vi "Add Device to Stack.vi"(8 "error in (no error)":errorcluster, 10 "Device in":refnum<class "Device.lvclass">, 11 "IP Connection in":refnum<class "IP Connection.lvclass">) -> (0 "error out":errorcluster, 2 "Device out":refnum<class "Device.lvclass">, 3 "IP Connection out":refnum<class "IP Connection.lvclass">)   [LabVIEW 2011, in "Tinkerforge.lvlib" / "IP Connection.lvclass"]
doc: "This VI adds <B>Device</B> to the stack."
uses:
  IP Connection.lvclass
  Device/Device.lvclass
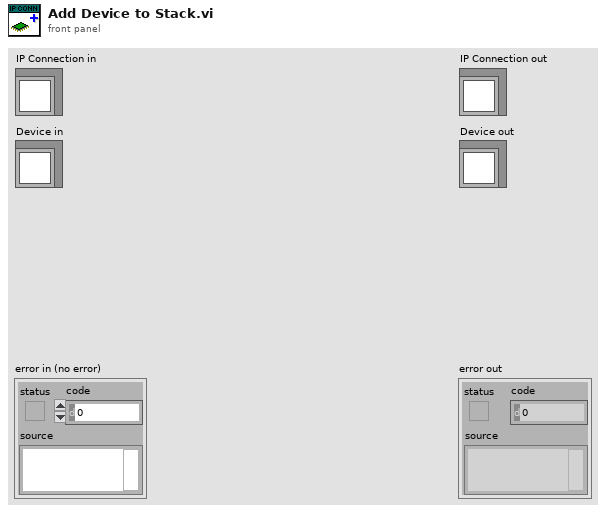
[diagram p1: front panel]
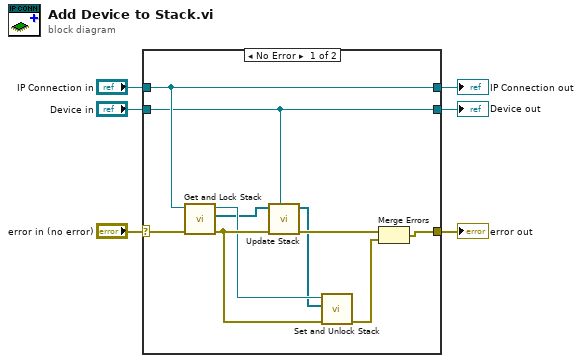
[diagram p0: block diagram]
diagram:
  n1 = case shown="No Error" "error in (no error)" {
    selector: "error in (no error)" -> [w14 w19]
    tunnel: [w16 w19] -> w5
    tunnel: [w13 w18] -> w3
    tunnel: "IP Connection in" -> [w13 w18]
    tunnel: "Device in" -> [w7 w17]
    tunnel: [w7 w17] -> w1
    frame No Error {
      n2 = call "Get and Lock Stack.vi"("error in (no error)"=w14, "IP Connection in"=w13) -> ("error out"=w12:errorcluster, "Stack"=w9:refnum<class "Device.lvclass">[], "IP Connection out"=w10:refnum<class "IP Connection.lvclass">)  [unwired: 7 in]
      n3 = call "Update Stack.vi"("Device"=w7, "error in (no error)"=w12, "Stack in"=w9) -> ("error out"=w15:errorcluster, "Stack out"=w8:refnum<class "Device.lvclass">[])  [unwired: 7 in]
      n4 = call "Set and Unlock Stack.vi"("error in (no error)"=w12, "Stack"=w8, "IP Connection in"=w10) -> ("error out"=w11:errorcluster)  [unwired: 7 in, 1 out]
      n5 = Merge Errors(w15, w11) -> (w16:errorcluster)
    }
    frame Error {
    }
  }
  "error out" <- w5
  "IP Connection out" <- w3
  "Device out" <- w1
